vi "conveyor-product.vi"(3 "COLOUR":T2, 4 "speed in":i32(listbox), 5 "Cluster":T1) -> (2 "Cluster o":T1)   [LabVIEW 2026]
uses:
  colour-radio-buton.ctl
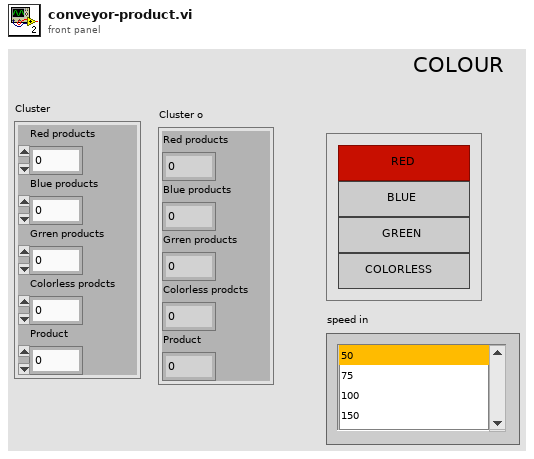
[diagram p1: front panel]
types:
  T1 = cluster{"Red products":u16, "Blue products":u16, "Grren products":u16, "Colorless prodcts":u16, "Product":u16}
  T2 = typedef "colour-radio-buton.ctl" = enum32{"RED", "BLUE", "GREEN", "colorless"}
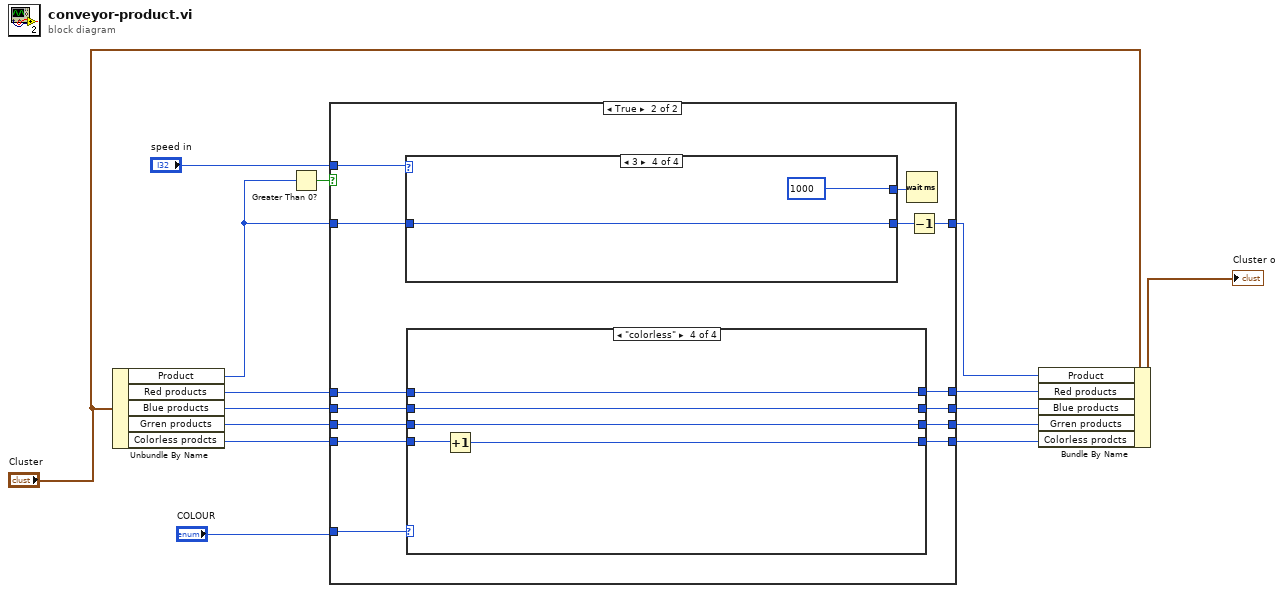
[diagram p0: block diagram]
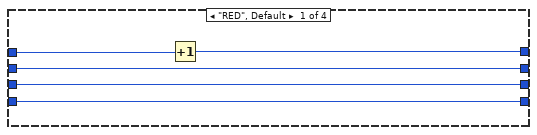
[diagram p3: hidden frame]
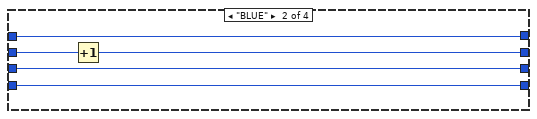
[diagram p4: hidden frame]
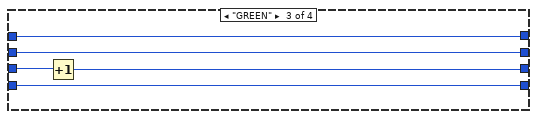
[diagram p5: hidden frame]
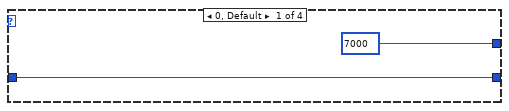
[diagram p6: hidden frame]
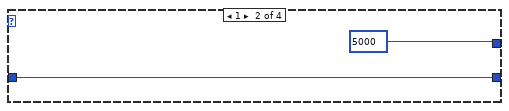
[diagram p7: hidden frame]
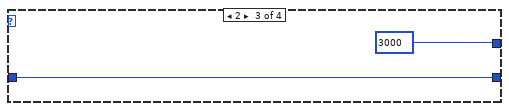
[diagram p8: hidden frame]
diagram:
  n1 = Unbundle By Name("Cluster") -> ("Product"=w15:u16, "Red products"=w12:u16, "Blue products"=w11:u16, "Grren products"=w10:u16, "Colorless prodcts"=w9:u16)
  n2 = Greater Than 0?(x=w15) -> (x > 0?=w14:bool)
  n3 = case shown="True" w14 {
    tunnel: w15 -> [w20 w33]
    tunnel: [w20 w21] -> w4
    tunnel: "speed in" -> [_ w34]
    tunnel: w12 -> [w19 w31]
    tunnel: w11 -> [w18 w29]
    tunnel: w10 -> [w17 w27]
    tunnel: w9 -> [w16 w25]
    tunnel: "COLOUR" -> [_ w32]
    tunnel: [w19 w30] -> w8
    tunnel: [w18 w28] -> w7
    tunnel: [w17 w26] -> w6
    tunnel: [w16 w24] -> w5
    frame False {
    }
    frame True {
      n4 = case shown="3" w34 {
        tunnel: w33 -> [w55 w58 w60 w62]
        tunnel: [w55 w58 w60 w62] -> w22
        tunnel: [u32 7000 ("milliseconds to wait") u32 5000 ("milliseconds to wait") u32 3000 ("milliseconds to wait") u32 1000 ("milliseconds to wait")] -> w23
        frame 0, Default {
        }
        frame 1 {
        }
        frame 2 {
        }
        frame 3 {
        }
      }
      n5 = case shown="\"colorless\"" w32 {
        tunnel: w31 -> [w39 w44 w49 w54]
        tunnel: [w38 w44 w49 w54] -> w30
        tunnel: w29 -> [w37 w41 w47 w53]
        tunnel: [w37 w40 w47 w53] -> w28
        tunnel: w27 -> [w36 w43 w46 w52]
        tunnel: [w36 w43 w45 w52] -> w26
        tunnel: w25 -> [w35 w42 w48 w51]
        tunnel: [w35 w42 w48 w50] -> w24
        frame "RED", Default {
          n6 = Increment(x=w39) -> (x+1=w38:u16)
        }
        frame "BLUE" {
          n7 = Increment(x=w41) -> (x+1=w40:u16)
        }
        frame "GREEN" {
          n8 = Increment(x=w46) -> (x+1=w45:u16)
        }
        frame "colorless" {
          n9 = Increment(x=w51) -> (x+1=w50:u16)
        }
      }
      n10 = Wait (ms)(milliseconds to wait=w23) -> ()  [unwired: 1 out]
      n11 = Decrement(x=w22) -> (x-1=w21:u16)
    }
  }
  n12 = Bundle By Name(cluster="Cluster", "Product"=w4, "Red products"=w8, "Blue products"=w7, "Grren products"=w6, "Colorless prodcts"=w5) -> (→"Cluster o":T1)
